vi "SP Show-Hide Markers.vi"(6 "Channel":i8=1 min=1 max=99 step=1, 7 "Plot References":refnum<vi>[](array[refnum]), 8 "error in (no error)":errorcluster, 9 "Show Markers":bool, 10 "Marker Values Ref":refnum<vi>, 11 "Plot Reference":refnum<vi>) -> (0 "error out":errorcluster)   [LabVIEW 2011]
uses:
  TypeDefs/SP Plot Cluster Object.ctl
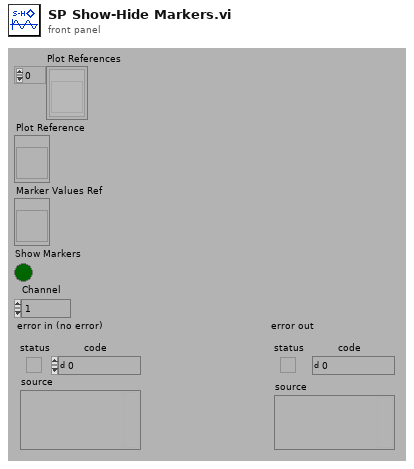
[diagram p1: front panel]
types:
  T1 = typedef "SP Plot Cluster Object.ctl" = enum16{"Plot", "CH Reference", "CH Label", "Start Label", "Stop Label", "Units Label", "Selected?", "CH Markers"}
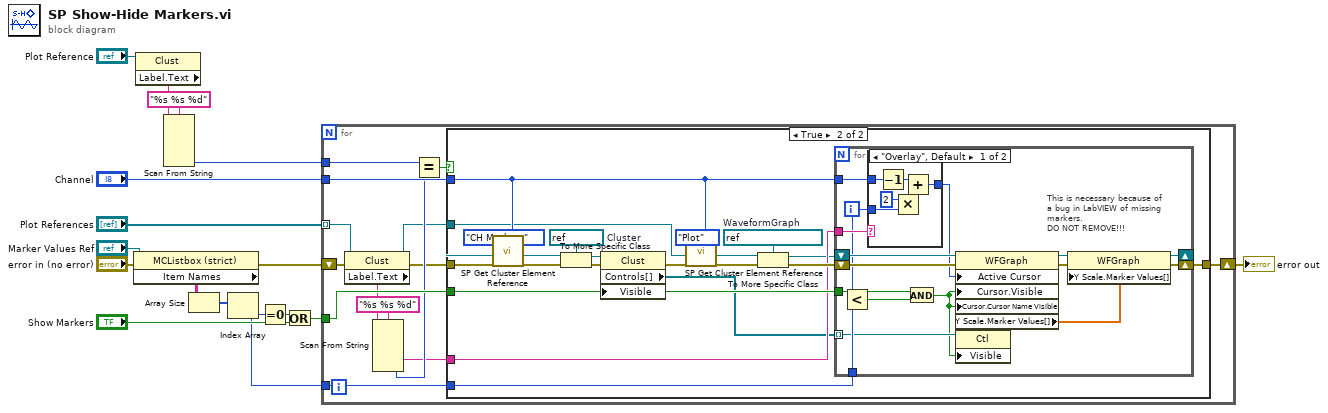
[diagram p0: block diagram]
diagram:
  n1 = property class="MCListbox (strict)"(reference="Marker Values Ref", error in="error in (no error)") -> (error out=w12:errorcluster, "Item Names"=w15:string[][])  [unwired: 1 out]
  n2 = property class="Clust"(reference="Plot Reference") -> ("Label.Text"=w7:string)  [unwired: 1 in, 2 out]
  n3 = Scan From String(format string="%s %s %d", input string=w7) -> (output 3=w3:i32)  [unwired: 2 in, 8 out]
  n4 = Array Size(array=w15) -> (size(s)=w14:i32[])
  n5 = Index Array(array=w14) -> (element=w1:i32)  [unwired: 1 in]
  n6 = Equal To 0?(x=w1) -> (x = 0?=w10:bool)
  n7 = Or(x=w10, y="Show Markers") -> (x .or. y?=w6:bool)
  n8 = for {
    tunnel: "Channel" -> [w30]
    tunnel: w6 -> [w28]
    shift-right: [w29] -> w11
    shift-left: w12 -> [w22]
    tunnel: "Plot References" -> [w24] mode=indexing
    tunnel: w3 -> [w20]
    tunnel: w1 -> [w17]
    n9 = property class="Clust"(reference=w24, error in=w22) -> (reference out=w23:refnum<vi>, error out=w21:errorcluster, "Label.Text"=w26:string)
    n10 = Scan From String(format string="%s %s %d", input string=w26) -> (output 2=w18:string, output 3=w27:i32)  [unwired: 2 in, 7 out]
    n11 = Equal?(x=w20, y=w27) -> (x = y?=w19:bool)
    n12 = case shown="True" w19 {
      tunnel: w30 -> [_ w46]
      tunnel: [w31 w49] -> w29
      tunnel: w28 -> [_ w48]
      tunnel: w23 -> [_ w45]
      tunnel: w21 -> [w31 w34]
      tunnel: w18 -> [_ w40]
      tunnel: w17 -> [_ w38]
      frame False {
      }
      frame True {
        w37 = refnum<vi> refnum  # Cluster
        w44 = refnum<vi> refnum  # WaveformGraph
        n13 = call "SP Get Cluster Element Reference.vi"("Channel"=w46, "Element"=SP_Plot_Cluster_Object."CH Markers", "Plot Reference"=w45) -> ("Element Reference"=w36:refnum<vi>)  [unwired: 6 out]
        n14 = To More Specific Class(target class=w37, reference=w36, error in=w34) -> (specific class reference=w35:refnum<vi>, error out=w33:errorcluster)
        n15 = property class="Clust"(reference=w35, error in=w33, "Visible"=w48) -> (error out=w43:errorcluster, "Controls[]"=w32:refnum<vi>[])  [unwired: 1 out]
        n16 = call "SP Get Cluster Element Reference.vi"("Channel"=w46, "Element"=SP_Plot_Cluster_Object."Plot", "Plot Reference"=w45) -> ("Element Reference"=w41:refnum<vi>)  [unwired: 6 out]
        n17 = To More Specific Class(target class=w44, reference=w41, error in=w43) -> (specific class reference=w39:refnum<vi>, error out=w42:errorcluster)
        n18 = for {
          tunnel: w40 -> [w66]
          tunnel: w46 -> [w65]
          shift-right: [w53] -> w49
          shift-left: w42 -> [w63]
          shift-right: [w51] -> _
          shift-left: w39 -> [w64]
          tunnel: w48 -> [w62]
          tunnel: w38 -> [w59]
          tunnel: w32 -> [w57] mode=indexing
          i -> [w60]
          # "This is necessary because of\na bug in LabVIEW of missing\nmarkers.\nDO NOT REMOVE!!!"
          n19 = Less?(x=w60, y=w59) -> (x < y?=w61:bool)
          n20 = case shown="\"Overlay\", Default" w66 {
            tunnel: w65 -> [w70 _]
            tunnel: w60 -> [w69 w73]
            tunnel: [w68 w73] -> w58
            frame "Overlay", Default {
              n21 = Decrement(x=w70) -> (x-1=w67:i8)
              n22 = Multiply(x=2, y=w69) -> (x*y=w72:i32)
              n23 = Add(x=w67, y=w72) -> (x+y=w68:i32)
            }
            frame "Split" {
            }
          }
          n24 = And(x=w62, y=w61) -> (x .and. y?=w56:bool)
          n25 = property class="WFGraph"(reference=w64, error in=w63, "Active Cursor"=w58, "Cursor.Visible"=w56, "Cursor.Cursor Name Visible"=w56) -> (reference out=w52:refnum<vi>, error out=w54:errorcluster, "Y Scale.Marker Values[]"=w55:dbl[])
          n26 = property class="Ctl"(reference=w57, "Visible"=w56) -> ()  [unwired: 1 in, 2 out]
          n27 = property class="WFGraph"(reference=w52, error in=w54, "Y Scale.Marker Values[]"=w55) -> (reference out=w51:refnum<vi>, error out=w53:errorcluster)
        }
      }
    }
  }
  "error out" <- w11
